vi "Demo.vi"() -> ()   [LabVIEW 2015]
uses:
  <vilib>/Utility/miscctls.llb/LVRowAndColumnTypeDef.ctl
  <vilib>/drjdpowell/SQLite Library/SQL Connection/Open (string).vi
  <vilib>/drjdpowell/SQLite Library/SQL Connection/Connection.lvclass
panel:
  out "Album ID":T1 caption="선택 시작"
  in  "Update":bool
  in  "Delete":bool
  in  "Artist":i64(ring) items=["Richard Wagner"=1, "Ludwig van Beethoven"=2, "Spongebob"=3, "Alen Walker"=4, "Mili"=5, "Steve Aoki & Yellow Claw"=6, "M2U x NICODE"=7]
  out "Data Display Center":string[][](table) caption="Database Albums"
  out "error out":errorcluster
  in  "New Artist":bool
  in  "Insert":bool
  in  "Album":string
  in  "STOP":bool
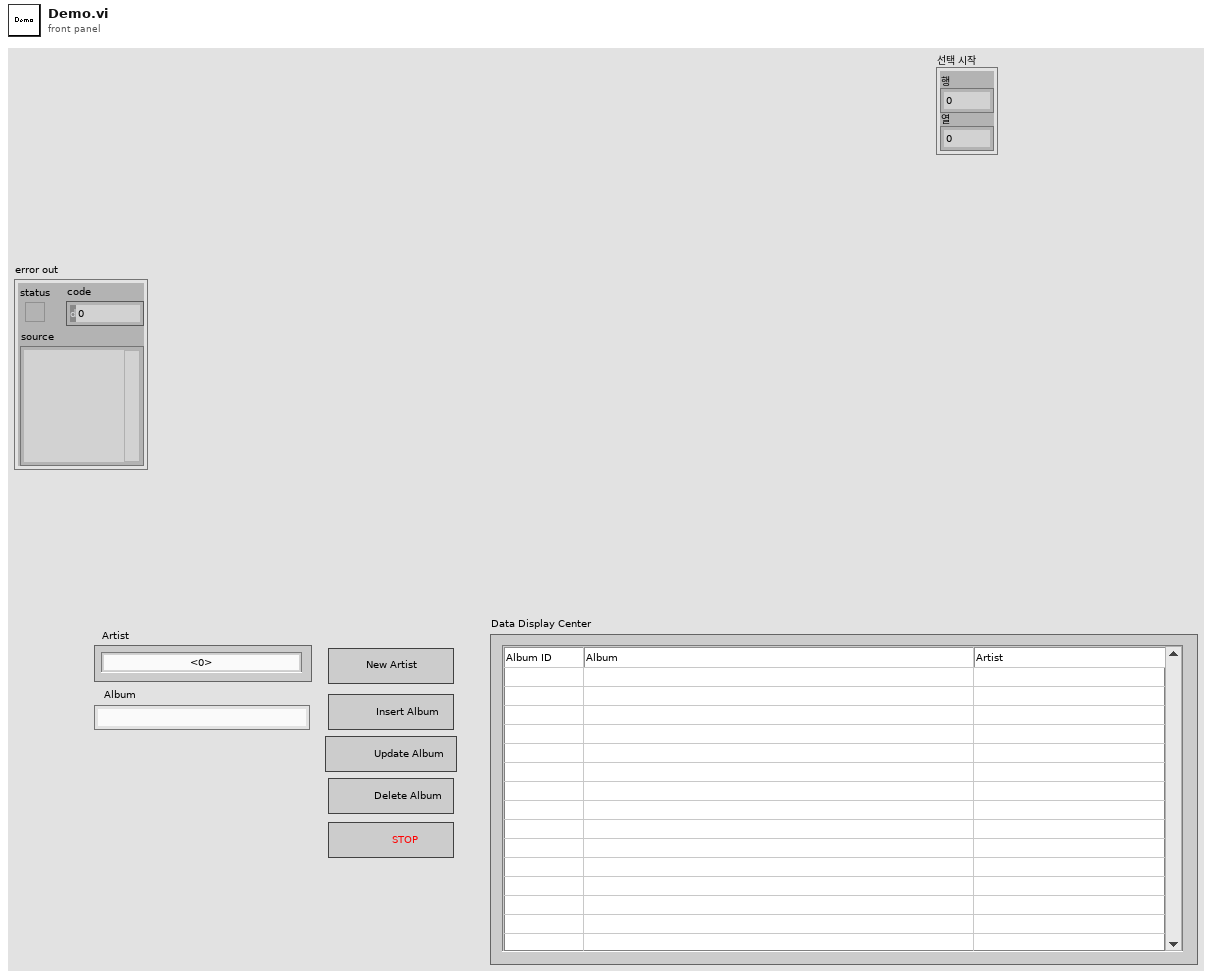
[diagram p1: front panel]
types:
  T1 = typedef "LVRowAndColumnTypeDef.ctl" = cluster{"Row":i32, "Column":i32}
  T2 = enum16{"Init", "Idle", "Read", "Insert", "Update", "Delete"}
  T3 = enum8{"Enabled", "Disabled", "Disabled and Grayed Out"}
  T4 = cluster{"Column:Get Column String":string, "Column:Get Column I64":i64}[]
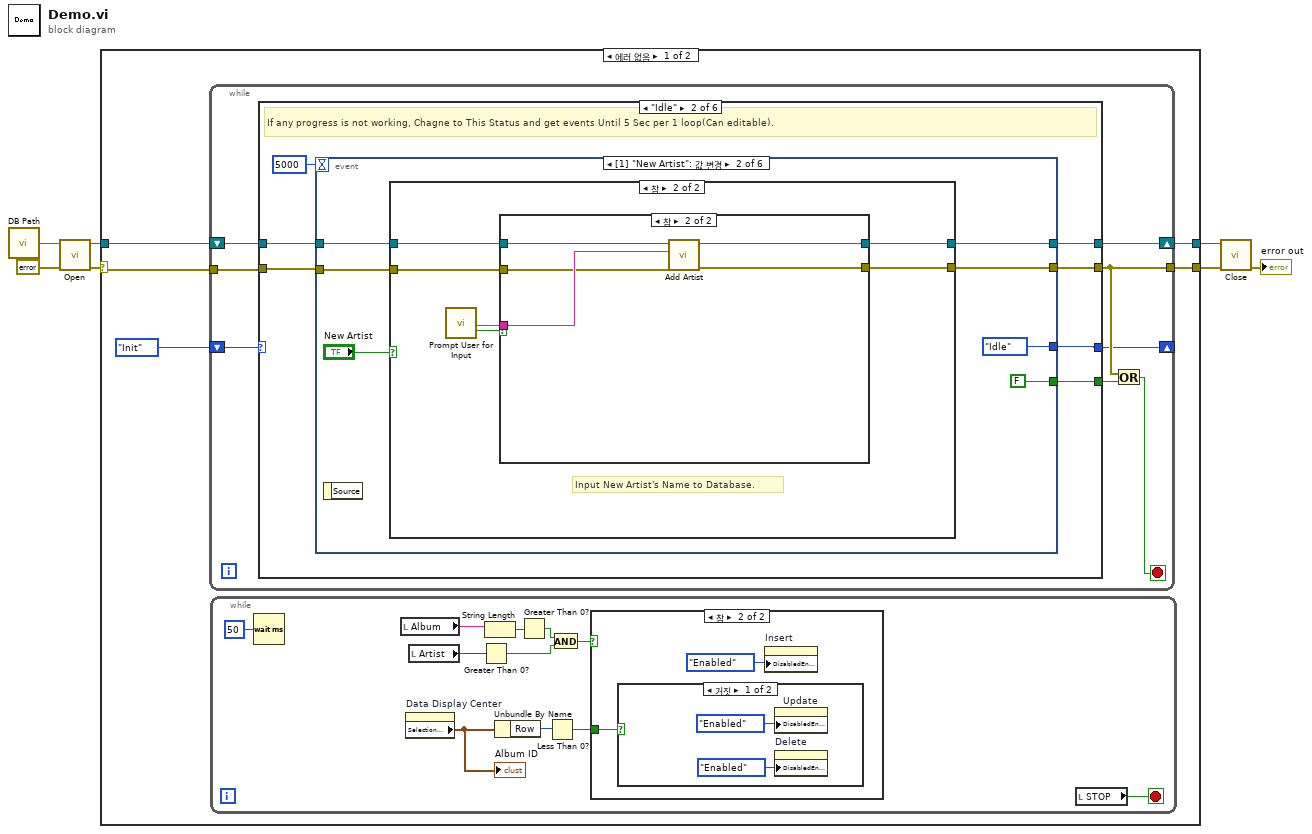
[diagram p0: block diagram]
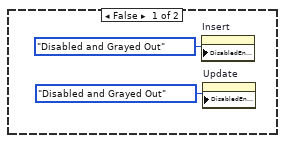
[diagram p2: hidden frame]
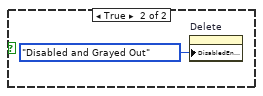
[diagram p3: hidden frame]
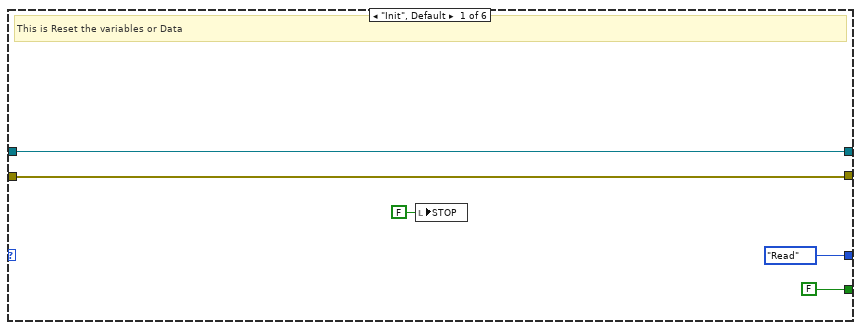
[diagram p4: hidden frame]
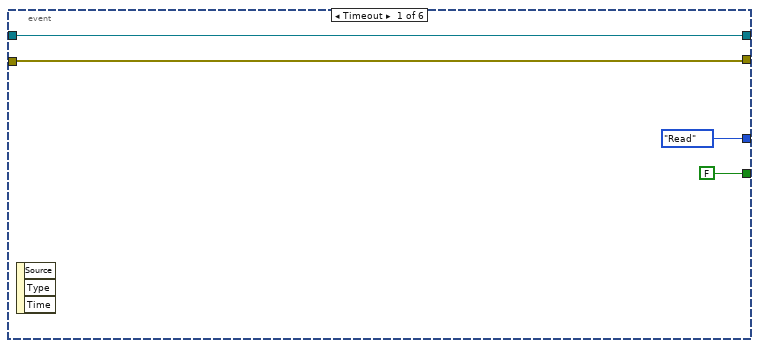
[diagram p5: hidden frame]
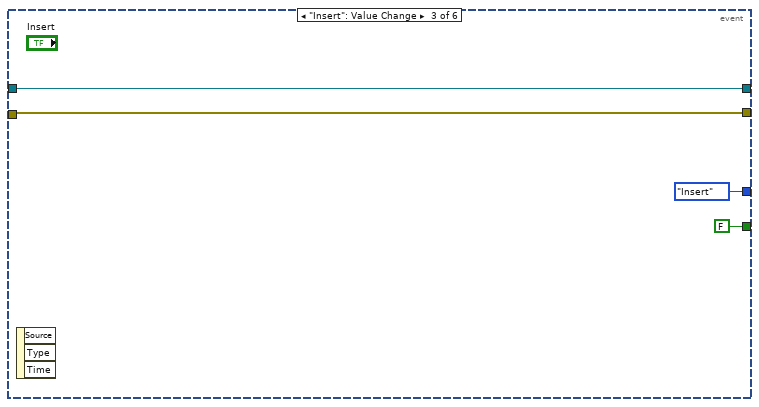
[diagram p8: hidden frame]
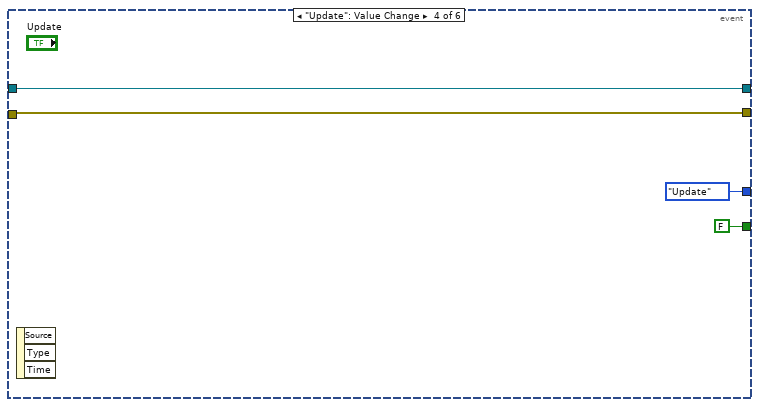
[diagram p9: hidden frame]
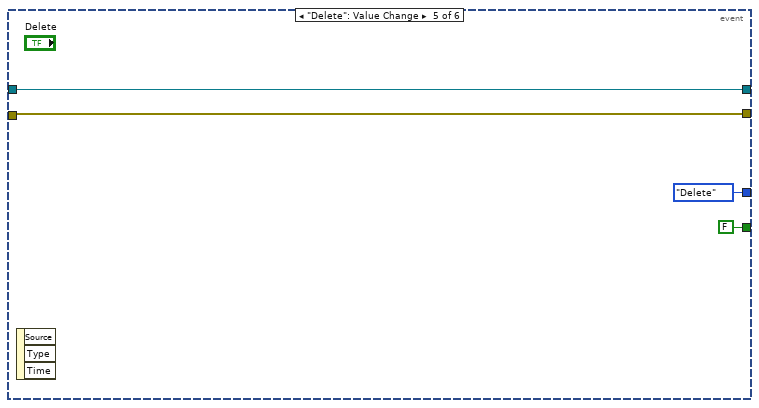
[diagram p10: hidden frame]
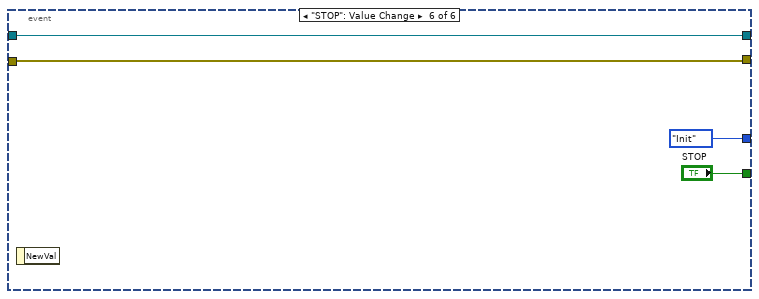
[diagram p11: hidden frame]
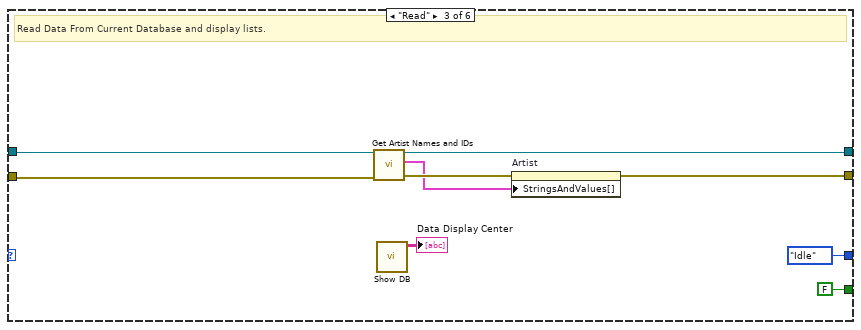
[diagram p12: hidden frame]
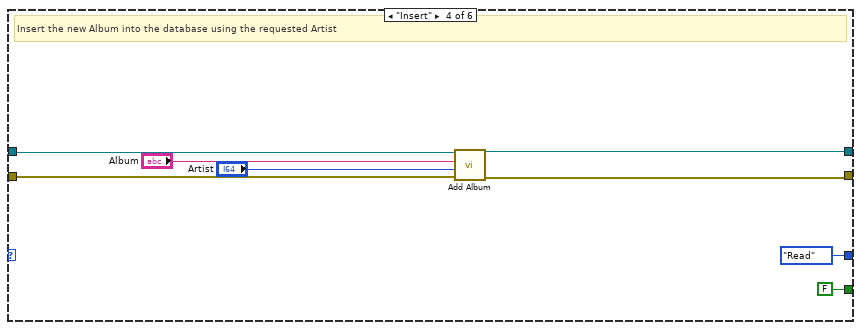
[diagram p13: hidden frame]
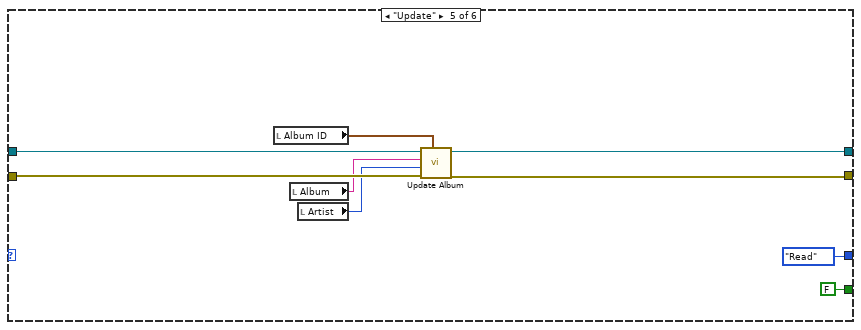
[diagram p14: hidden frame]
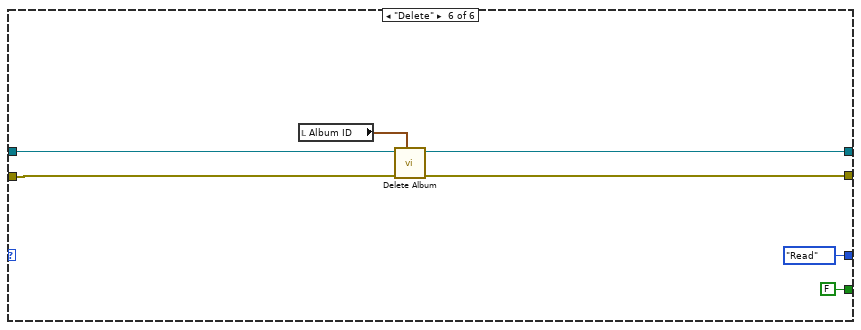
[diagram p15: hidden frame]
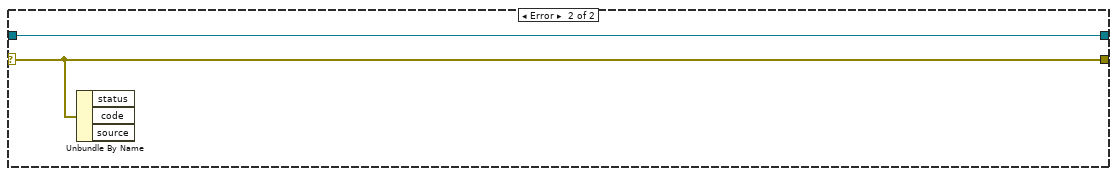
[diagram p16: hidden frame]
diagram:
  n1 = call "DB Path.vi"() -> ("DB Path"=w7:string)
  n2 = call-poly <vilib>:"Open.vi"("error in (no error)"=errorcluster {"status"=FALSE, "code"=0, "source"=""}, "db file"=w7) -> ("error out"=w4:errorcluster, "SQLite Connection"=w6:refnum<class "Connection.lvclass">)  [unwired: 8 in]
  n3 = case shown="에러 없음" w4 {
    selector: w4 -> [w10 w126]
    tunnel: [w9 w126] -> w3
    tunnel: w6 -> [w12 w127]
    tunnel: [w11 w127] -> w5
    frame No Error {
      n4 = while {
        shift-right: [w36] -> w11
        shift-left: w12 -> [w38]
        tunnel: w10 -> [w37]
        tunnel: [w34] -> w9
        shift-right: [w31] -> _
        shift-left: T2."Init" -> [w35]
        stop <- w32 stop-if-true
        n5 = case shown="\"Idle\"" w35 {
          tunnel: w38 -> [w41 w46 w97 w105 w116 w125]
          tunnel: w37 -> [w40 w45 w96 w106 w115 w124]
          tunnel: [w41 w48 w95 w108 w114 w123] -> w36
          tunnel: [w40 w47 w94 w107 w113 w122] -> w34
          tunnel: [FALSE ("stop") w49 FALSE ("stop") FALSE ("stop") FALSE ("stop") FALSE ("stop")] -> w33
          tunnel: [T2."Read" w50 T2."Idle" T2."Read" T2."Read" T2."Read"] -> w31
          frame "Init", Default {
            # "This is Reset the variables or Data"
            n6 = local write "STOP"(FALSE ("STOP")) -> ()
          }
          frame "Idle" {
            # "If any progress is not working, Chagne to This Status and get events Until 5 Sec per 1 loop(Can editable)."
            n7 = event shown="[1] \"New Artist\": 값 변경" {
              selector: _ -> [_ _ _ _ _ _]
              dyn-events: _ -> [_ _ _ _ _ _]
              timeout: 5000 -> [_ _ _ _ _ _]
              tunnel: [FALSE ("stop") FALSE ("stop") FALSE ("STOP") FALSE ("STOP") FALSE ("STOP") "STOP"] -> w49
              tunnel: [T2."Read" T2."Idle" T2."Insert" T2."Update" T2."Delete" T2."Init"] -> w50
              tunnel: [w52 w56 w79 w82 w86 w90] -> w48
              tunnel: [w51 w55 w78 w81 w85 w89] -> w47
              tunnel: w46 -> [w52 w58 w79 w82 w86 w90]
              tunnel: w45 -> [w51 w57 w78 w81 w85 w89]
              event Timeout {
                n8 = event-data() -> ()  [unwired: 1 in, 3 out]
              }
              event "New Artist": Value Change {
                n9 = event-data() -> ()  [unwired: 1 in, 1 out]
                n10 = case shown="참" "New Artist" {
                  tunnel: w58 -> [w63 w67]
                  tunnel: w57 -> [w62 w66]
                  tunnel: [w63 w65] -> w56
                  tunnel: [w62 w64] -> w55
                  frame False {
                  }
                  frame True {
                    # "Input New Artist's Name to Database."
                    n11 = call "Prompt User for Input"() -> ("Name"=w68:string, "OK"=w69:bool)  [unwired: 17 in, 1 out]
                    n12 = case shown="참" w69 {
                      tunnel: w68 -> [_ w76]
                      tunnel: w67 -> [w71 w75]
                      tunnel: w66 -> [w70 w74]
                      tunnel: [w71 w73] -> w65
                      tunnel: [w70 w72] -> w64
                      frame False {
                      }
                      frame True {
                        n13 = call "Add Artist.vi"("error in (no error)"=w74, "Artist Name"=w76, "SQLite Connection in"=w75) -> ("error out"=w72:errorcluster, "SQLite Connection out"=w73:refnum<class "Connection.lvclass">)  [unwired: 7 in]
                      }
                    }
                  }
                }
              }
              event "Insert": Value Change {
                n14 = event-data() -> ()  [unwired: 1 in, 3 out]
              }
              event "Update": Value Change {
                n15 = event-data() -> ()  [unwired: 1 in, 3 out]
              }
              event "Delete": Value Change {
                n16 = event-data() -> ()  [unwired: 1 in, 3 out]
              }
              event "STOP": Value Change {
                n17 = event-data() -> ()  [unwired: 1 in, 1 out]
              }
            }
          }
          frame "Read" {
            # "Read Data From Current Database and display lists."
            n18 = call "Get Artist Names and IDs.vi"("error in (no error)"=w96, "SQLite Connection in"=w97) -> ("error out"=w98:errorcluster, "배열"=w93:T4, "SQLite Connection out"=w95:refnum<class "Connection.lvclass">)  [unwired: 7 in]
            n19 = call "Show DB.vi"() -> ("Result Set"=→"Data Display Center":string[][])  [unwired: 11 in]
            n20 = property on="Artist" class="Ring (엄격한)"(error in=w98, "StringsAndValues[]"=w93) -> (error out=w94:errorcluster)  [unwired: 1 in, 1 out]
          }
          frame "Insert" {
            # "Insert the new Album into the database using the requested Artist"
            n21 = call "Add Album.vi"("error in (no error)"=w106, "Artist ID"="Artist", "Name"="Album", "SQLite Connection in"=w105) -> ("error out"=w107:errorcluster, "SQLite Connection out"=w108:refnum<class "Connection.lvclass">)  [unwired: 6 in]
          }
          frame "Update" {
            n22 = local read "Album ID"() -> (w110:T1)
            n23 = local read "Album"() -> (w112:string)
            n24 = local read "Artist"() -> (w111:i64)
            n25 = call "Update Album.vi"("Album ID"=w110, "error in (no error)"=w115, "Artist ID"=w111, "Name"=w112, "SQLite Connection in"=w116) -> ("error out"=w113:errorcluster, "SQLite Connection out"=w114:refnum<class "Connection.lvclass">)  [unwired: 5 in]
          }
          frame "Delete" {
            n26 = local read "Album ID"() -> (w121:T1)
            n27 = call "Delete Album.vi"("Album ID"=w121, "error in (no error)"=w124, "SQLite Connection in"=w125) -> ("error out"=w122:errorcluster, "SQLite Connection out"=w123:refnum<class "Connection.lvclass">)  [unwired: 7 in]
          }
        }
        n28 = Or(x=w34, y=w33) -> (x .or. y?=w32:bool)
      }
      n29 = while {
        stop <- w17 stop-if-true
        n30 = Wait (ms)(milliseconds to wait=u32 50 ("대기 시간(ms)")) -> ()  [unwired: 1 out]
        n31 = local read "Album"() -> (w19:string)
        n32 = property on="Data Display Center" class="Tbl (엄격한)"() -> ("Selection Start"=w13:T1)  [unwired: 2 in, 2 out]
        "Album ID" <- w13
        n33 = local read "Artist"() -> (w18:i64)
        n34 = Greater Than 0?(x=w18) -> (x > 0?=w21:bool)
        n35 = String Length(string=w19) -> (length=w23:i32)
        n36 = Unbundle By Name(w13) -> ("Row"=w14:i32)
        n37 = Greater Than 0?(x=w23) -> (x > 0?=w22:bool)
        n38 = Less Than 0?(x=w14) -> (x < 0?=w15:bool)
        n39 = And(x=w22, y=w21) -> (x .and. y?=w20:bool)
        n40 = case shown="참" w20 {
          tunnel: w15 -> [_ w26]
          frame False {
            n41 = property on="Insert" class="Bool"("DisabledEnum"=T3."Disabled and Grayed Out" ("비활성화")) -> ()  [unwired: 2 in, 2 out]
            n42 = property on="Update" class="Bool"("DisabledEnum"=T3."Disabled and Grayed Out" ("비활성화")) -> ()  [unwired: 2 in, 2 out]
          }
          frame True {
            n43 = case shown="거짓" w26 {
              frame False {
                n44 = property on="Update" class="Bool"("DisabledEnum"=T3."Enabled" ("비활성화")) -> ()  [unwired: 2 in, 2 out]
                n45 = property on="Delete" class="Bool"("DisabledEnum"=T3."Enabled" ("비활성화")) -> ()  [unwired: 2 in, 2 out]
              }
              frame True {
                n46 = property on="Delete" class="Bool"("DisabledEnum"=T3."Disabled and Grayed Out" ("비활성화")) -> ()  [unwired: 2 in, 2 out]
              }
            }
            n47 = property on="Insert" class="Bool"("DisabledEnum"=T3."Enabled" ("비활성화")) -> ()  [unwired: 2 in, 2 out]
          }
        }
        n48 = local read "STOP"() -> (w17:bool)
      }
    }
    frame Error {
      n49 = Unbundle By Name(w126) -> ()  [unwired: 3 out]
    }
  }
  n50 = call-dynamic "Close.vi"("error in (no error)"=w3, "SQLite Connection in"=w5) -> ("error out"=→"error out":errorcluster)  [unwired: 9 in]
